vi "Actor Core.vi"(8 "error in":errorcluster, 11 "ConfigurableActor in":refnum<class "ConfigurableActor.lvclass">) -> (0 "error out":errorcluster, 3 "Actor out":refnum<class "Actor.lvclass">)   [LabVIEW 2014, in "ConfigurableActor.lvclass"]
doc: "(<B>Filename</B>: Actor Framework.lvlib:Actor.lvclass:Actor Core.vi)\n\nReceives messages to the actor, reacts to them, and initiates any error handling that may shut the actor down.\n\nDescendant classes may override this VI to append parallel tasks for the actor to complete while it handles messages. Overrides use the Call Parent Method node."
uses:
  ConfigurableActor.lvclass
  <vilib>/ActorFramework/Actor/Actor.lvclass
  ConfigurableActor.lvclass/ConfigurableActor.ctl
  <vilib>/ActorFramework/Actor/Actor.lvclass/Actor.ctl
  <vilib>/ActorFramework/Message Enqueuer/Message Enqueuer.lvclass/Message Enqueuer.ctl
  <vilib>/ActorFramework/Message Enqueuer/Init from Existing Queue.vi
  <vilib>/ActorFramework/Message Enqueuer/Enqueue.vi
  <vilib>/ActorFramework/Message Priority Queue/Priority Enqueue.vi
  <vilib>/ActorFramework/Message Enqueuer/Message Enqueuer.lvclass
  <vilib>/ActorFramework/Stop Msg/Stop Msg.lvclass
panel:
  out "data":errorcluster
  out "Fully Qualified Name":string
  in  "Launch Nested Actor":bool
  # "Actor UI"
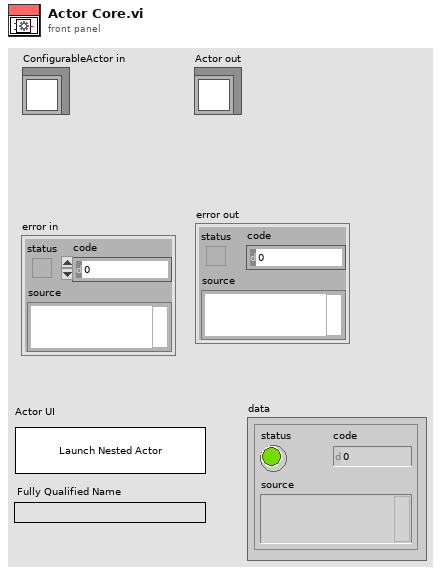
[diagram p1: front panel]
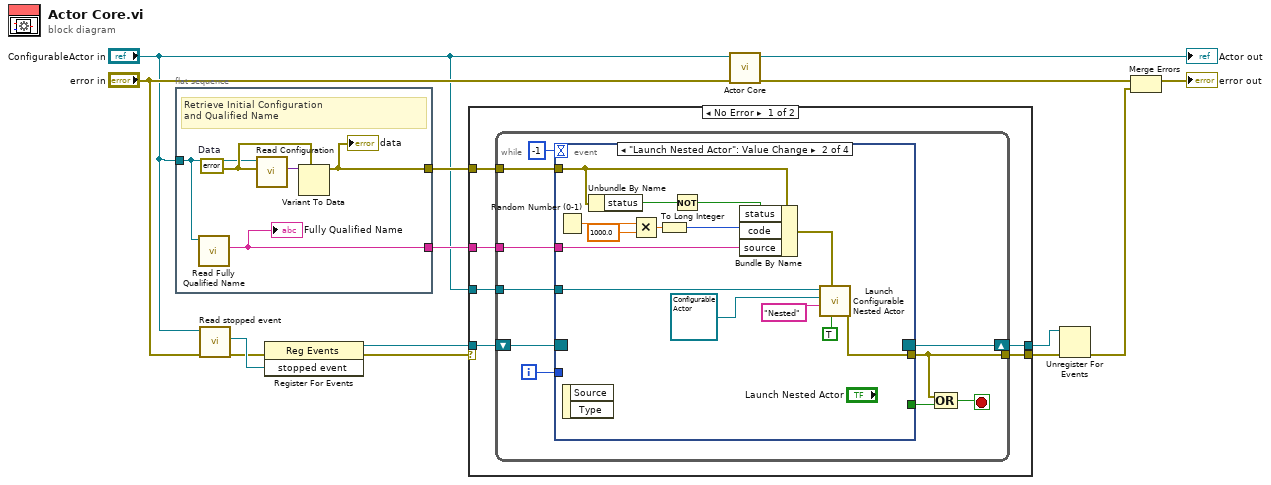
[diagram p0: block diagram]
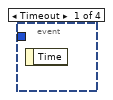
[diagram p2: hidden frame]
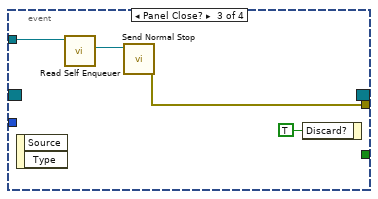
[diagram p3: hidden frame]
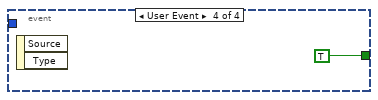
[diagram p4: hidden frame]
diagram:
  n1 = flat-sequence {
    tunnel: [w16] -> w7
    tunnel: [w17] -> w6
    tunnel: "ConfigurableActor in" -> [w15]
    frame #0 {
      w18 = errorcluster {"status"=FALSE, "code"=0, "source"=""}  # Data
      # "Retrieve Initial Configuration\nand Qualified Name"
      n2 = call "Read Fully Qualified Name.vi"("ConfigurableActor in"=w15) -> ("Fully Qualified Name"=w17:string)  [unwired: 8 in, 2 out]
      "Fully Qualified Name" <- w17
      n3 = call "Read Configuration.vi"("Type"=w18, "ConfigurableActor in"=w15) -> ("value"=w19:variant)  [unwired: 5 in, 4 out]
      n4 = Variant To Data(type=w18, Variant=w19) -> (data=w16:errorcluster)  [unwired: 1 in, 1 out]
      "data" <- w16
    }
  }
  n5 = call "Read stopped event.vi"("error in (no error)"="error in", "ConfigurableActor in"="ConfigurableActor in") -> ("error out"=w3:errorcluster, "stopped event"=w9:refnum<user-event>)  [unwired: 7 in, 1 out]
  n6 = register-events(error in=w3, w9) -> (reference out=w1:refnum<event-registration>, error out=w2:errorcluster)  [unwired: 1 in]
  n7 = case shown="No Error" w2 {
    selector: w2 -> [_ w56]
    tunnel: w1 -> [w25 w55]
    tunnel: [w24 w55] -> w13
    tunnel: [w23 w56] -> w12
    tunnel: w7 -> [w22 _]
    tunnel: w6 -> [w21 _]
    tunnel: "ConfigurableActor in" -> [w20 _]
    frame No Error {
      n8 = while {
        tunnel: w20 -> [w33]
        tunnel: [w31] -> w23
        shift-right: [w32] -> w24
        shift-left: w25 -> [w34]
        tunnel: w22 -> [w27]
        tunnel: w21 -> [w26]
        i -> [w28]
        stop <- w30 stop-if-true
        n9 = event shown="[1] \"Launch Nested Actor\": Value Change" {
          selector: w34 -> [_ _ _ _]
          dyn-events: [_ _ _ _] -> w32
          timeout: -1 -> [_ _ _ _]
          tunnel: w33 -> [_ w49 w52 _]
          tunnel: [_ w47 w50 _] -> w31
          tunnel: [_ _ _ TRUE] -> w29
          tunnel: w28 -> [_ _ _ _]
          tunnel: w27 -> [_ w39 _ _]
          tunnel: w26 -> [_ w45 _ _]
          event Timeout {
            n10 = event-data() -> ()  [unwired: 1 in, 1 out]
          }
          event "Launch Nested Actor": Value Change {
            n11 = Random Number (0-1)() -> (number: 0 to 1=w43:dbl)
            n12 = event-data() -> ()  [unwired: 1 in, 2 out]
            n13 = Unbundle By Name(w39) -> ("status"=w38:bool)
            n14 = Multiply(x=w43, y=1000.0) -> (x*y=w41:dbl)
            n15 = To Long Integer(number=w41) -> (32bit integer=w40:i32)
            n16 = Not(x=w38) -> (.not. x?=w37:bool)
            n17 = Bundle By Name(cluster=w39, "status"=w37, "code"=w40, "source"=w45) -> (w44:errorcluster)
            n18 = call "Launch Configurable Nested Actor.vi"("Open Actor Core front panel? (F)"=TRUE, "Configuration"=w44, "Name"="Nested", "Configurable Dependency"=refnum<class "ConfigurableActor.lvclass"> refnum ("ConfigurableActor.lvclass"), "Actor"=w49) -> ("error out"=w47:errorcluster)  [unwired: 6 in]
          }
          event Panel Close? {
            n19 = event-data() -> ()  [unwired: 1 in, 2 out]
            n20 = call <vilib>:"Read Self Enqueuer.vi"("Actor"=w52) -> ("Self Enqueuer"=w51:refnum<class "Message Enqueuer.lvclass">)  [unwired: 10 in]
            n21 = call <vilib>:"Send Normal Stop.vi"("Message Enqueuer"=w51) -> ("error out"=w50:errorcluster)  [unwired: 10 in]
            n22 = event-data("Discard?"=TRUE) -> ()  [unwired: 1 in, 1 out]
          }
          event User Event {
            n23 = event-data() -> ()  [unwired: 1 in, 2 out]
          }
        }
        n24 = Compound Arithmetic op=OR(w31, w29) -> (w30:bool)
      }
    }
    frame Error {
    }
  }
  n25 = call-parent "Actor Core.vi"("error in"="error in", "Actor in"="ConfigurableActor in") -> ("error out"=w10:errorcluster, "Actor out"=→"Actor out":refnum<class "Actor.lvclass">)  [unwired: 8 in]
  n26 = Unregister For Events(event registration refnum=w13, error in=w12) -> (error out=w8:errorcluster)
  n27 = Merge Errors(w10, w8) -> (→"error out":errorcluster)
